vi "SPI_Set_Clock.vi"(2 "ClockDivisor":u32 max=65535 step=1, 3 "Handle":u32) -> (0 "ClockFrequency":u32, 1 "FTC_status":u32)   [LabVIEW 2010]
uses:
  WINNT/system32/FTCSPI.dll
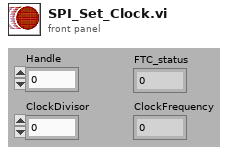
[diagram p1: front panel]
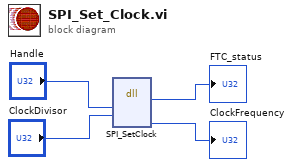
[diagram p0: block diagram]
diagram:
  n1 = dll-call lib="C:/Users/WINNT/system32/FTCSPI.dll" fn="SPI_SetClock"("Handle"="Handle", "ClockDivisor"="ClockDivisor") -> ("FTC_status"=→"FTC_status":u32, "ClockFrequency"=→"ClockFrequency":u32)  [unwired: 6 in, 2 out]
